vi "Create_Bin_Indices.vi"(2 "No Of Bins":i32, 3 "Cycle Start TIme":dbl[](array[numeric]) format="%.2f") -> (0 "Bin Number":i32[](array[numeric]), 1 "Bin Start Time":dbl[](array[numeric]))   [LabVIEW 2011]
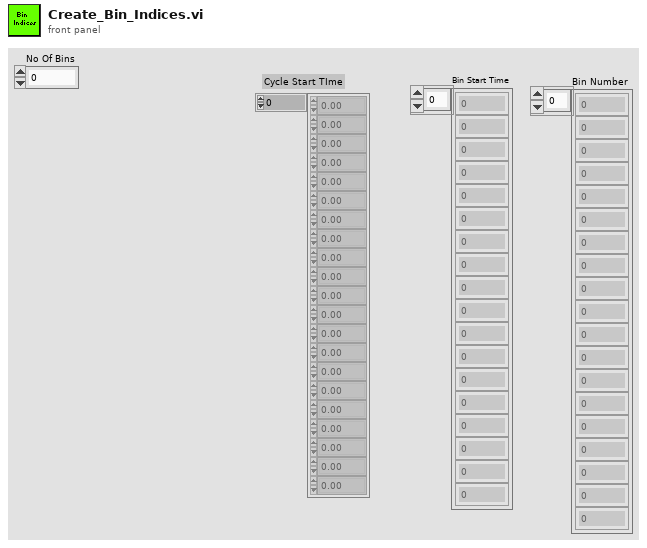
[diagram p1: front panel]
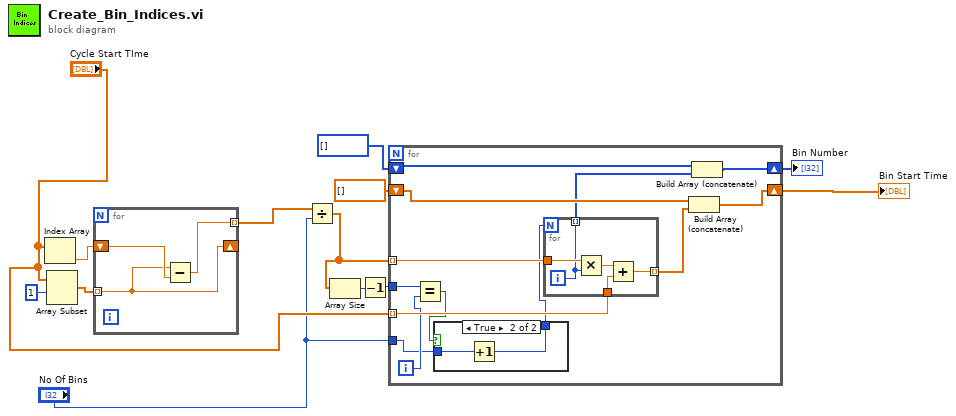
[diagram p0: block diagram]
diagram:
  n1 = Index Array(array="Cycle Start TIme") -> (element=w12:dbl)  [unwired: 1 in]
  n2 = Array Subset(array="Cycle Start TIme", index=1) -> (w11:dbl[])  [unwired: 1 in]
  n3 = for {
    shift-right: [w14] -> _
    shift-left: w12 -> [w16]
    tunnel: w11 -> [w14] mode=indexing
    tunnel: [w15] -> w10 mode=indexing
    n4 = Subtract(x=w14, y=w16) -> (x-y=w15:dbl)
  }
  n5 = Divide(x=w10, y="No Of Bins") -> (x/y=w5:dbl[])
  n6 = Array Size(array=w5) -> (size(s)=w7:i32)
  n7 = Decrement(x=w7) -> (x-1=w6:i32)
  n8 = for {
    tunnel: w5 -> [w29] mode=indexing
    tunnel: "Cycle Start TIme" -> [w28] mode=indexing
    shift-right: [w25] -> w3
    shift-left: dbl[] [] -> [w26]
    tunnel: "No Of Bins" -> [w21]
    tunnel: w6 -> [w23]
    shift-right: [w17] -> w2
    shift-left: i32[] [] -> [w18]
    i -> [w24]
    n9 = Equal?(x=w23, y=w24) -> (x = y?=w22:bool)
    n10 = case shown="True" w22 {
      tunnel: w21 -> [w30 w32]
      tunnel: [w30 w31] -> w20
      frame False {
      }
      frame True {
        n11 = Increment(x=w32) -> (x+1=w31:i32)
      }
    }
    n12 = for {
      N: w20 -> [_]
      tunnel: w29 -> [w37]
      tunnel: w28 -> [w35]
      tunnel: [w34] -> w27 mode=indexing
      tunnel: [w33] -> w19 mode=indexing
      i -> [w33]
      n13 = Multiply(x=w37, y=w33) -> (x*y=w36:dbl)
      n14 = Add(x=w36, y=w35) -> (x+y=w34:dbl)
    }
    n15 = Build Array (concatenate)(w26, w27) -> (w25:dbl[])
    n16 = Build Array (concatenate)(w18, w19) -> (w17:i32[])
  }
  "Bin Start Time" <- w3
  "Bin Number" <- w2
